vi "oldEnemyTeamToOOEnemyTeam.vi"(5 "Side":enum16{"Esquerdo", "Direito"}(ring), 7 "Team":enum16{"Azul", "Amarelo"}(ring), 8 "error in (no error)":errorcluster, 10 "enemy_robots":T1[](array[typedef]), 11 "Enemy in":refnum<class "Enemy.lvclass">) -> (0 "error out":errorcluster, 3 "Enemy out":refnum<class "Enemy.lvclass">)   [LabVIEW 2023, in "Enemy.lvclass"]
uses:
  Enemy.lvclass
  Robot_class/Robot.lvclass
  Vision_class/Old vision/Controls/AI Robot.ctl
  Vision_class/Old vision/Controls/Functions Enum.ctl
  Vision_class/Old vision/Controls/AttackerStates.ctl
  Vision_class/Old vision/Controls/PathDests.ctl
  Vision_class/Old vision/Controls/PathDest.ctl
  Game_class/Navigation/VSSNavigation/VSSAttackerStates.ctl
  Team_class/Team.lvclass/Team.ctl
  Object_class/Object.lvclass/Object.ctl
  Robot_class/Robot.lvclass/Robot.ctl
  Object_class/Write x.vi
  Object_class/Write y.vi
  Robot_class/Write orientation.vi
  Robot_class/Write id.vi
  Robot_class/Write est_v_tang.vi
  Robot_class/Write est_v_norm.vi
  Team_class/Read RobotRef.vi
  Team_class/Write RobotRef.vi
panel:
  in  "Robot":refnum<class "Robot.lvclass">
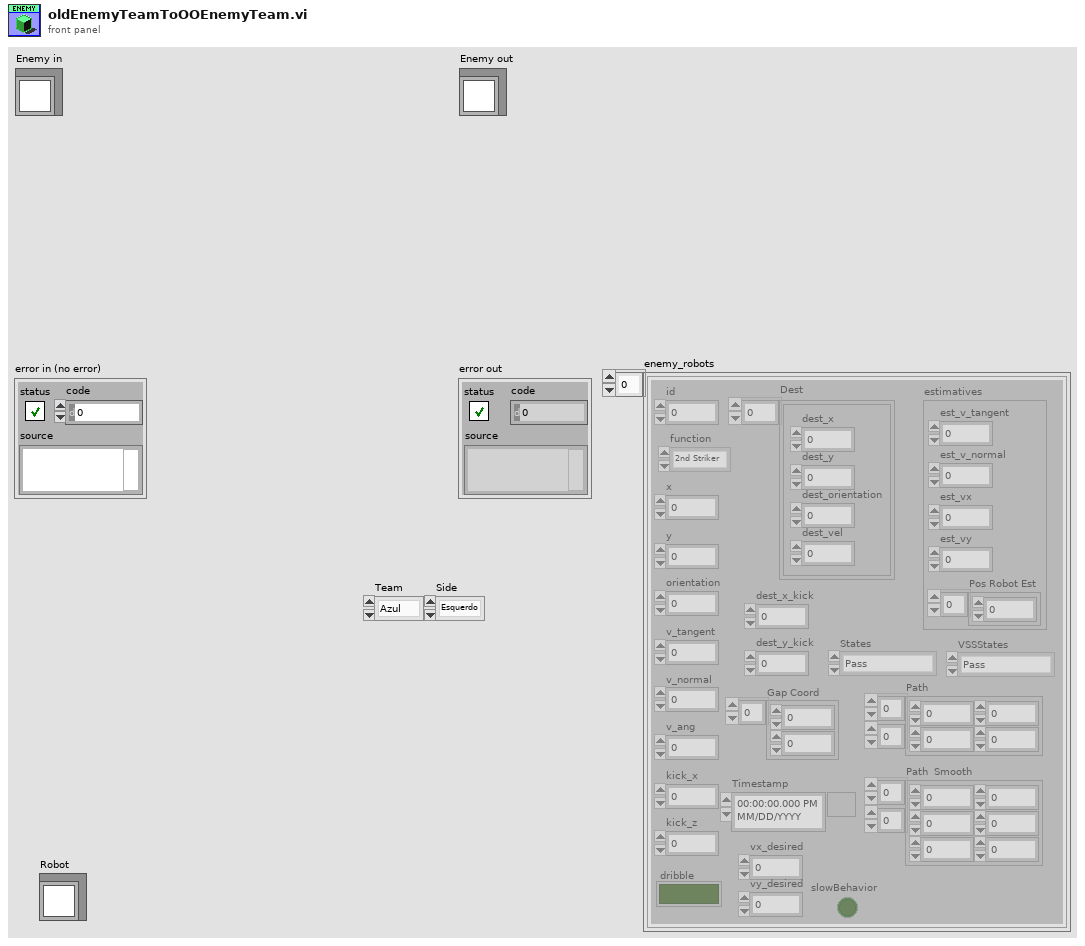
[diagram p1: front panel]
types:
  T1 = typedef "AI Robot.ctl" = cluster{"id":u32, "function":T2, "x":dbl, "y":dbl, "orientation":dbl, "v_tangent":dbl, "v_normal":dbl, "v_ang":dbl, "kick_x":dbl, "kick_z":dbl, "dribble":bool, "Timestamp":timestamp, "estimatives":cluster{"est_v_tangent":dbl, "est_v_normal":dbl, "est_vx":dbl, "est_vy":dbl, "Pos Robot Est":dbl[]}, "dest_x_kick":dbl, "dest_y_kick":dbl, "Gap Coord":dbl[], "States":T3, "Path ":dbl[][], "Path  Smooth":dbl[][], "Dest":T4, "vx_desired":dbl, "vy_desired":dbl, "slowBehavior":bool, "VSSStates":T6}
  T2 = typedef "Functions Enum.ctl" = enum16{"2nd Striker", "Attacker", "Goalie", "Defender", "Striker", "Goto 0", "Dummy", "Kicker", "ZigZag 0", "ZigZag 1", "ZigZag 2", "ZigZag 3", "ZigZag 4", "ZigZag 5", "ZigZag 6", "ZigZag 7", "ZigZag 8", ""}
  T3 = typedef "AttackerStates.ctl" = enum16{"Pass", "GoToTangent", "BallGetting", "GoToKick", ""}
  T4 = typedef "PathDests.ctl" = T5[]
  T5 = typedef "PathDest.ctl" = cluster{"dest_x":dbl, "dest_y":dbl, "dest_orientation":dbl, "dest_vel":dbl}
  T6 = typedef "VSSAttackerStates.ctl" = enum16{"Pass", "GoToTangent", "BallGetting", "GoToKick", "Rotate anti-clockwise", "Rotate Clockwise", ""}
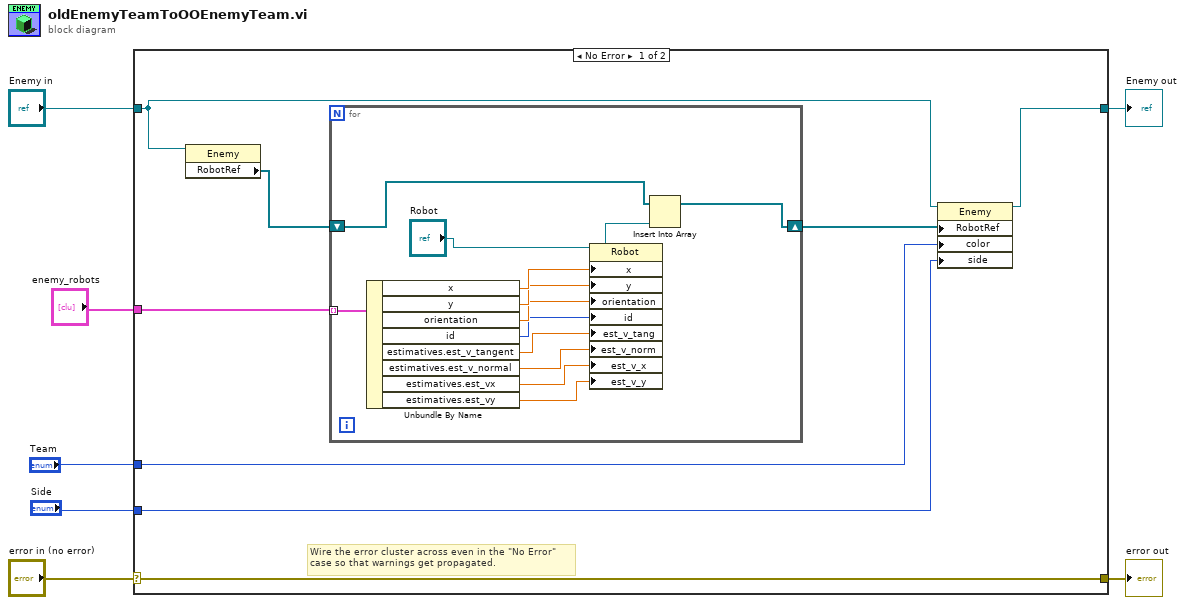
[diagram p0: block diagram]
diagram:
  n1 = case shown="No Error" "error in (no error)" {
    selector: "error in (no error)" -> [w15 w30]
    tunnel: [w15 w30] -> w6
    tunnel: [w12 w29] -> w4
    tunnel: "Enemy in" -> [w10 w29]
    tunnel: "enemy_robots" -> [w11 _]
    tunnel: "Team" -> [w14 _]
    tunnel: "Side" -> [w13 _]
    frame No Error {
      # "Wire the error cluster across even in the \"No Error\"\ncase so that warnings get propagated."
      n2 = property class="Enemy"(reference=w10) -> ("RobotRef"=w9:refnum<class "Robot.lvclass">[])  [unwired: 1 in, 2 out]
      n3 = for {
        shift-right: [w26] -> w8
        shift-left: w9 -> [w24]
        tunnel: w11 -> [w25] mode=indexing
        n4 = Unbundle By Name(w25) -> ("x"=w23:dbl, "y"=w22:dbl, "orientation"=w21:dbl, "id"=w20:u32, "estimatives.est_v_tangent"=w19:dbl, "estimatives.est_v_normal"=w18:dbl, "estimatives.est_vx"=w17:dbl, "estimatives.est_vy"=w16:dbl)
        n5 = property class="Robot"(reference="Robot", "x"=w23, "y"=w22, "orientation"=w21, "id"=w20, "est_v_tang"=w19, "est_v_norm"=w18, "est_v_x"=w17, "est_v_y"=w16) -> (reference out=w27:refnum<class "Robot.lvclass">)  [unwired: 1 in, 1 out]
        n6 = Insert Into Array(array=w24, new element=w27) -> (w26:refnum<class "Robot.lvclass">[])  [unwired: 1 in]
      }
      n7 = property class="Enemy"(reference=w10, "RobotRef"=w8, "color"=w14, "side"=w13) -> (reference out=w12:refnum<class "Enemy.lvclass">)  [unwired: 1 in, 1 out]
    }
    frame Error {
    }
  }
  "error out" <- w6
  "Enemy out" <- w4
